vi "Intercept.vi"(0 "Y":dbl, 1 "X":dbl, 3 "X2":dbl, 4 "XY":dbl, 7 "N":dbl) -> (5 "Intercept":dbl)   [LabVIEW 2012]
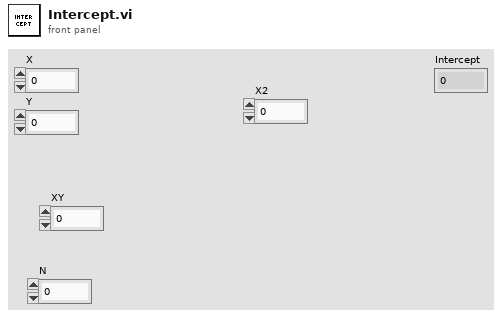
[diagram p1: front panel]
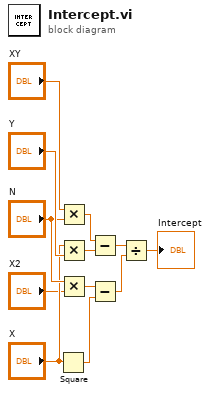
[diagram p0: block diagram]
diagram:
  n1 = Square(x="X") -> (x^2=w5:dbl)
  n2 = Multiply(x="XY", y="N") -> (x*y=w10:dbl)
  n3 = Multiply(x="X", y="Y") -> (x*y=w9:dbl)
  n4 = Multiply(x="N", y="X2") -> (x*y=w4:dbl)
  n5 = Subtract(x=w10, y=w9) -> (x-y=w8:dbl)
  n6 = Subtract(x=w4, y=w5) -> (x-y=w3:dbl)
  n7 = Divide(x=w8, y=w3) -> (x/y=→"Intercept":dbl)
